vi "Configure Parameter to Measure.vi"(8 "error in (no error)":errorcluster, 10 "Sparameters (string)":string[](array[string]), 11 "VNA-Keysight PNA in":refnum<class "VNA-Keysight PNA.lvclass">) -> (0 "error out":errorcluster, 3 "VNA-Keysight PNA out":refnum<class "VNA-Keysight PNA.lvclass">)   [LabVIEW 2020, in "VNA-Keysight PNA.lvclass"]
uses:
  VNA-Keysight PNA.lvclass
  C:/Sandbox/RF Bench/Source Code/WiSpry Test Framework/Instruments/Instrument.lvclass
  Instrument.lvclass/Instrument.ctl
  Instrument.lvclass
  <instrlib>/Keysight PNA Series/Keysight PNA Series.lvlib
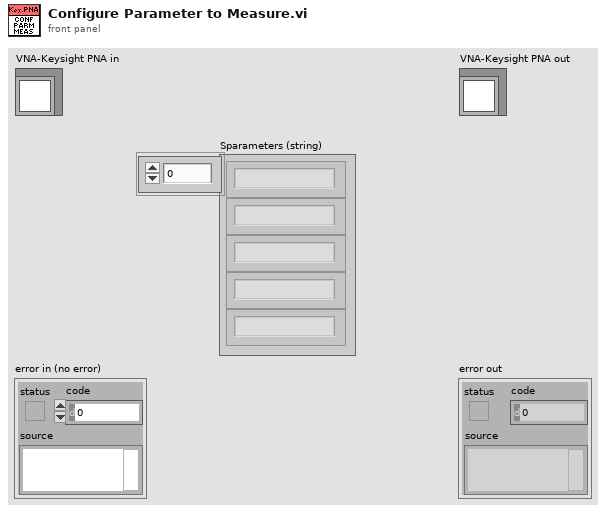
[diagram p1: front panel]
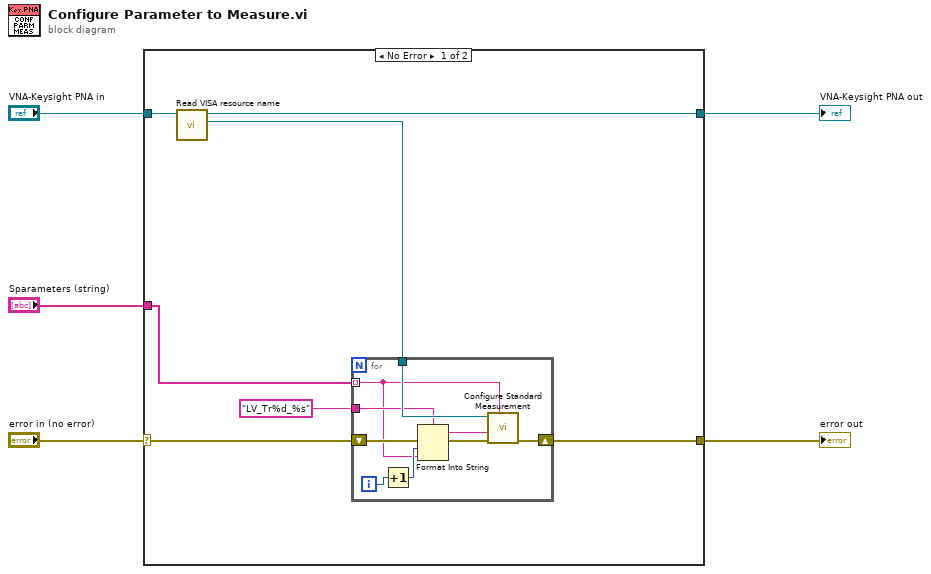
[diagram p0: block diagram]
diagram:
  n1 = case shown="No Error" "error in (no error)" {
    selector: "error in (no error)" -> [w10 w22]
    tunnel: [w11 w23] -> w3
    tunnel: "VNA-Keysight PNA in" -> [w12 w23]
    tunnel: [w9 w22] -> w2
    tunnel: "Sparameters (string)" -> [w8 _]
    frame No Error {
      n2 = call "Read VISA resource name.vi"("Instrument in"=w12) -> ("VISA resource name"=w7:refnum<visa-resource-name>, "Instrument out"=w11:refnum<class "VNA-Keysight PNA.lvclass">)  [unwired: 9 in]
      n3 = for {
        shift-right: [w21] -> w9
        shift-left: w10 -> [w19]
        tunnel: w8 -> [w13] mode=indexing
        tunnel: w7 -> [w20]
        tunnel: "LV_Tr%d_%s" -> [w14]
        i -> [w18]
        n4 = Increment(x=w18) -> (x+1=w17:i32)
        n5 = Format Into String(format string=w14, error in=w19, w17, w13) -> (resulting string=w15:string, error out=w16:errorcluster)  [unwired: 1 in]
        n6 = call <instrlib>:"Configure Standard Measurement.vi"("Measurement Parameters (S11)"=w13, "error in (no error)"=w16, "Measurement Name (CH1_S11_1)"=w15, "VISA resource name"=w20) -> ("error out"=w21:errorcluster)  [unwired: 6 in, 1 out]
      }
    }
    frame Error {
    }
  }
  "error out" <- w2
  "VNA-Keysight PNA out" <- w3
